vi "LaunchReentrantVI.vi"(5 "rcm file path":path, 7 "datum":T1, 8 "error in (no error)":errorcluster, 10 "item name in":string, 11 "vi reference in":refnum<vi>) -> (0 "error out":errorcluster, 3 "vi reference out":refnum<vi>)   [LabVIEW 2009]
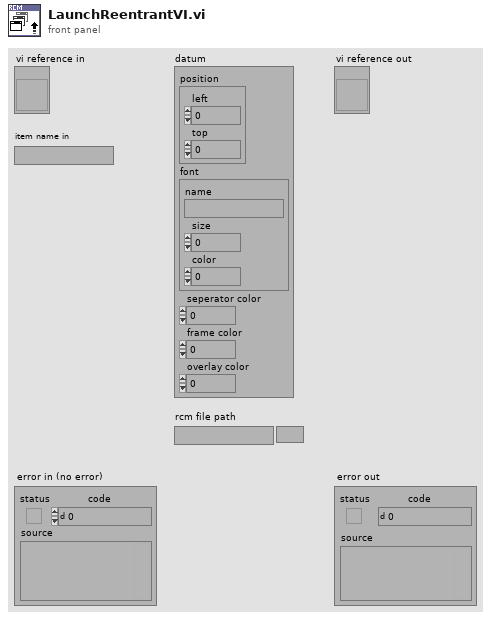
[diagram p1: front panel]
types:
  T1 = cluster{"position":cluster{"left":u32, "top":u32}, "font":cluster{"name":string, "size":i16, "color":u32}, "seperator color":u32, "frame color":u32, "overlay color":u32}
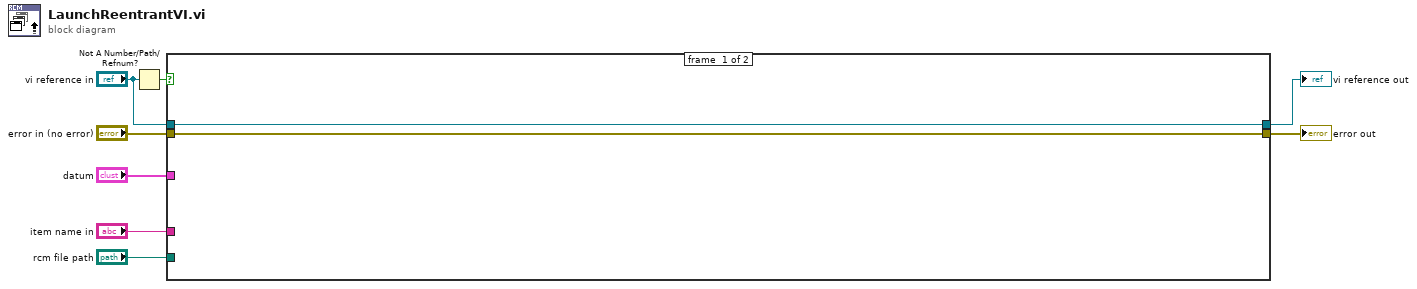
[diagram p0: block diagram]
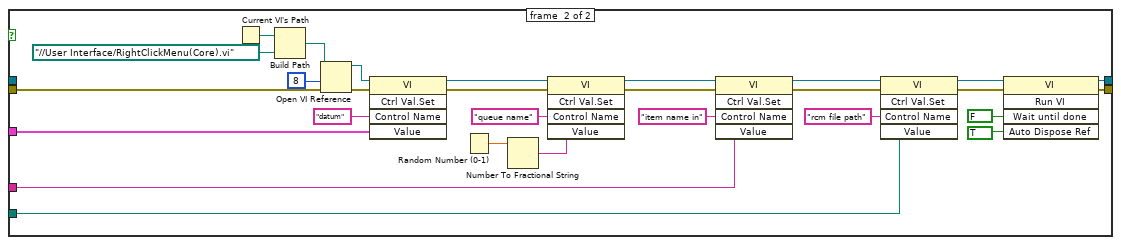
[diagram p2: hidden frame]
diagram:
  n1 = Not A Number/Path/Refnum?(number/path/refnum="vi reference in") -> (NaN/Path/Refnum?=w7:bool)
  n2 = case shown="True" w7 {
    tunnel: "datum" -> [_ w34]
    tunnel: [w10 w25] -> w6
    tunnel: "vi reference in" -> [w10 _]
    tunnel: [w9 w24] -> w4
    tunnel: "error in (no error)" -> [w9 w27]
    tunnel: "item name in" -> [_ w15]
    tunnel: "rcm file path" -> [_ w14]
    frame #0 {
    }
    frame #1 {
      n3 = Current VI's Path() -> (path=w12:path)
      n4 = Build Path(base path=w12, name or relative path=path "../../User Interface/RightClickMenu(Core).vi" ("vi path")) -> (appended path=w11:path)
      n5 = Open VI Reference(vi path=w11, options=8, error in (no error)=w27) -> (vi reference=w32:refnum<vi>, error out=w31:errorcluster)  [unwired: 3 in]
      n6 = invoke class="VI" method="Ctrl Val.Set"(reference=w32, error in=w31, "Control Name"="datum", "Value"=w34) -> (reference out=w30:refnum<vi>, error out=w29:errorcluster)  [unwired: 1 in, 3 out]
      n7 = Random Number (0-1)() -> (number: 0 to 1=w33:dbl)
      n8 = Number To Fractional String(number=w33) -> (F-format string=w26:string)  [unwired: 3 in]
      n9 = invoke class="VI" method="Ctrl Val.Set"(reference=w30, error in=w29, "Control Name"="queue name", "Value"=w26) -> (reference out=w21:refnum<vi>, error out=w16:errorcluster)  [unwired: 1 in, 3 out]
      n10 = invoke class="VI" method="Ctrl Val.Set"(reference=w21, error in=w16, "Control Name"="item name in", "Value"=w15) -> (reference out=w20:refnum<vi>, error out=w17:errorcluster)  [unwired: 1 in, 3 out]
      n11 = invoke class="VI" method="Ctrl Val.Set"(reference=w20, error in=w17, "Control Name"="rcm file path", "Value"=w14) -> (reference out=w19:refnum<vi>, error out=w18:errorcluster)  [unwired: 1 in, 3 out]
      n12 = invoke class="VI" method="Run VI"(reference=w19, error in=w18, "Wait until done"=FALSE ("Wait Until Done"), "Auto Dispose Ref"=TRUE ("Auto Dispose Reference")) -> (reference out=w25:refnum<vi>, error out=w24:errorcluster)  [unwired: 1 in, 3 out]
    }
  }
  "vi reference out" <- w6
  "error out" <- w4
